vi "ZLIB File Information__ogtk.vi"(0 "file path":path, 1 "encode MacBinary (F)":bool, 3 "error in (no error)":errorcluster) -> (4 "created macbinary":bool, 5 "file timestamp":u32, 6 "file path out":path, 7 "directory":bool, 8 "file attributes":u32, 9 "error out":errorcluster)   [LabVIEW 2011]
doc: "Retrives specific information for a disk file preparing a Mac resource files as MACBIN data file fork."
panel:
  # "Please visit http://www.OpenG.org to learn about the\nOpen Source LabVIEW software movement.\n\nNOTICE -- YOU MUST LEAVE THIS NOTICE IN PLACE.  PER THE TERMS OF THE LICENSE BELOW, YOU MAY SUBLICENSE THIS SOFTWARE \nIN ANY WAY THAT DOES NOT CONFLICT WITH THIS LICENSE.\n\n### BSD License (http://www.opensource.org/licenses/bsd-license.php) Begin ###\n \nCopyright (C) 2008 Rolf Kalbermatter rolf.kalbermatter@citeng.com\n\nAll rights reserved.\n\nRedistribution and use in source and binary forms, with or without modification, are permitted provided that the following conditions are met:\n\n    * Redistributions of source code must retain the above copyright notice, this list of conditions and the following disclaimer.\n    * Redistributions in binary form must reproduce the above copyright notice, this list of conditions and the following disclaimer in the \n       documentation and/or other materials provided with the distribution.\n    * Neither the name of SciWare, James Kring, Inc., nor the names of its contributors may be used to endorse or promote products derived \n       from this software without specific prior written permission.\n\nTHIS SOFTWARE IS PROVIDED BY THE COPYRIGHT HOLDERS AND CONTRIBUTORS \"AS IS\" AND ANY EXPRESS OR IMPLIED WARRANTIES, \nINCLUDING, BUT NOT LIMITED TO, THE IMPLIED WARRANTIES OF MERCHANTABILITY AND FITNESS FOR A PARTICULAR PURPOSE ARE \nDISCLAIMED. IN NO EVENT SHALL THE COPYRIGHT OWNER OR CONTRIBUTORS BE LIABLE FOR ANY DIRECT, INDIRECT, INCIDENTAL,\n SPECIAL, EXEMPLARY, OR CONSEQUENTIAL DAMAGES (INCLUDING, BUT NOT LIMITED TO, PROCUREMENT OF SUBSTITUTE GOODS OR \nSERVICES; LOSS OF USE, DATA, OR PROFITS; OR BUSINESS INTERRUPTION) HOWEVER CAUSED AND ON ANY THEORY OF LIABILITY, \nWHETHER IN CONTRACT, STRICT LIABILITY, OR TORT (INCLUDING NEGLIGENCE OR OTHERWISE) ARISING IN ANY WAY OUT OF THE USE \nOF THIS SOFTWARE, EVEN IF ADVISED OF THE POSSIBILITY OF SUCH DAMAGE.\n\n### BSD License End ###"
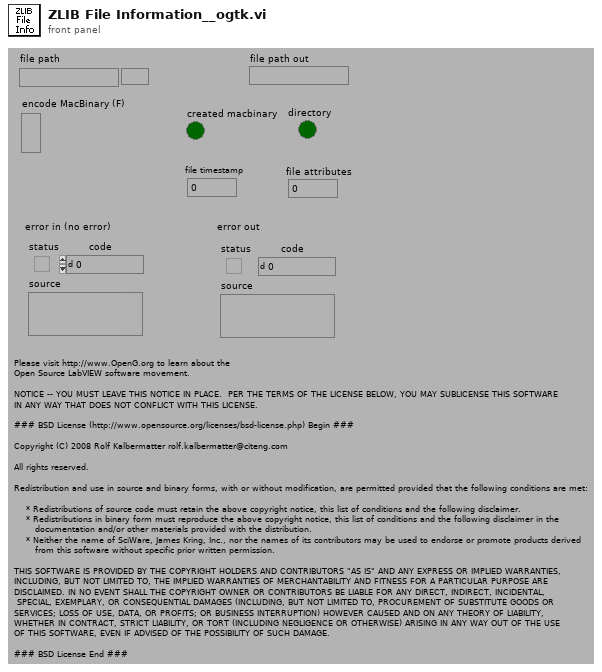
[diagram p1: front panel]
types:
  T1 = typedef "MACBIN Resource Header__ogtk.ctl" = cluster{"type":string, "creator":string, "data size":u32, "res size":u32, "creation date":u32, "mod date":u32, "finder flags":u16, "vertical pos":i16, "horizontal pos":i16, "finder id":u16, "script id":u8, "ext finder flags":u8}
  T2 = typedef "Librarian File Info Out.ctl" = cluster{"creation date":u32, "last mod date":u32, "type":string, "creator":string, "LV version":i32, "size":i32, "top level":bool}
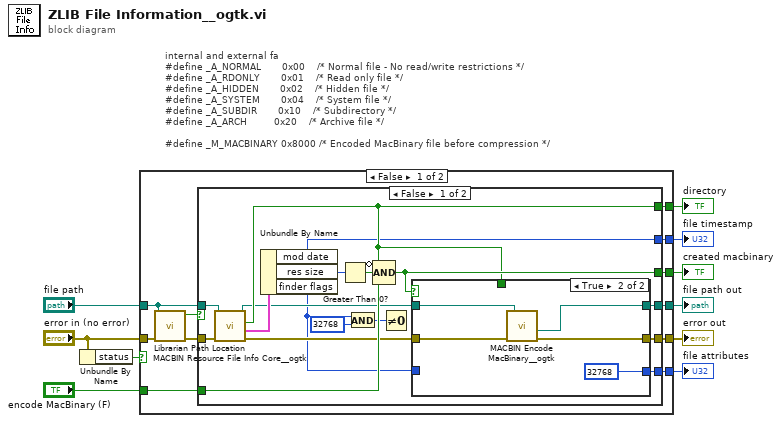
[diagram p0: block diagram]
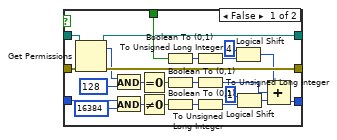
[diagram p2: hidden frame]
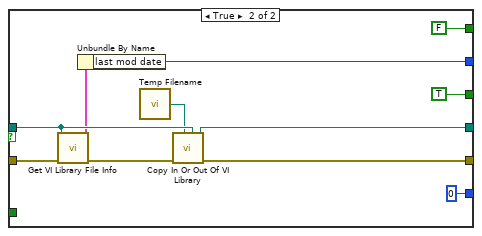
[diagram p3: hidden frame]
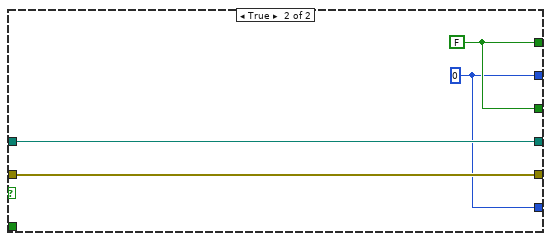
[diagram p4: hidden frame]
diagram:
  # "internal and external fa\n#define _A_NORMAL       0x00    /* Normal file - No read/write restrictions */\n#define _A_RDONLY       0x01    /* Read only file */\n#define _A_HIDDEN       0x02    /* Hidden file */\n#define _A_SYSTEM       0x04    /* System file */\n#define _A_SUBDIR       0x10    /* Subdirectory */\n#define _A_ARCH         0x20    /* Archive file */\n\n#define _M_MACBINARY 0x8000 /* Encoded MacBinary file before compression */"
  n1 = Unbundle By Name("error in (no error)") -> ("status"=w3:bool)
  n2 = case shown="False" w3 {
    tunnel: "file path" -> [w11 w82]
    tunnel: [w15 w79] -> w9
    tunnel: [w16 w80] -> w8
    tunnel: "error in (no error)" -> [w14 w81]
    tunnel: [w21 w82] -> w6
    tunnel: [w20 w81] -> w5
    tunnel: [w19 w79] -> w4
    tunnel: [w18 w80] -> w2
    tunnel: "encode MacBinary (F)" -> [w17 _]
    frame False {
      n3 = call <vilib>:"Librarian Path Location.vi"("error in (no error)"=w14, "path"=w11) -> ("error out"=w13:errorcluster, "path is in a VI library"=w12:bool)  [unwired: 5 in, 3 out]
      n4 = case shown="False" w12 {
        tunnel: w13 -> [w38 w77]
        tunnel: [w37 w71] -> w21
        tunnel: [w36 w72] -> w20
        tunnel: [w35 u32 0 ("Input")] -> w19
        tunnel: [w34 TRUE] -> w18
        tunnel: w17 -> [w33 _]
        tunnel: w11 -> [w32 w76]
        tunnel: [w31 FALSE ("is directory")] -> w16
        tunnel: [w29 w73] -> w15
        frame False {
          n5 = call <userlib>:"MACBIN Resource File Info Core__ogtk.vi"("error in (no error)"=w38, "resource file"=w32) -> ("error out"=w25:errorcluster, "file info out"=w30:T1, "is directory"=w31:bool, "resource file out"=w26:path)  [unwired: 3 in, 1 out]
          n6 = Unbundle By Name(w30) -> ("mod date"=w29:u32, "res size"=w28:u32, "finder flags"=w24:u16)
          n7 = Greater Than 0?(x=w28) -> (x > 0?=w27:bool)
          n8 = And(x=w24, y=u16 32768) -> (x .and. y?=w22:u16)
          n9 = Compound Arithmetic op=AND(invert w31, w27, w33) -> (w34:bool)
          n10 = Not Equal To 0?(x=w22) -> ()  [unwired: 1 out]
          n11 = case shown="True" w34 {
            tunnel: [w55 w67] -> w37
            tunnel: [w54 w66] -> w36
            tunnel: w26 -> [w56 w64]
            tunnel: w25 -> [w57 w63]
            tunnel: [w62 u32 32768 ("Input")] -> w35
            tunnel: w31 -> [w59 _]
            tunnel: w24 -> [w46 _]
            frame False {
              n12 = Get Permissions(8:w57, 11:w56) -> (0:w54:errorcluster, 3:w55:path, 5:w49:i16)  [unwired: 2 out]
              n13 = And(x=w49, y=i16 128) -> (x .and. y?=w53:i16)
              n14 = And(x=w46, y=u16 16384) -> (x .and. y?=w48:u16)
              n15 = Equal To 0?(x=w53) -> (x = 0?=w52:bool)
              n16 = Not Equal To 0?(x=w48) -> (x != 0?=w58:bool)
              n17 = Boolean To (0,1)(Boolean=w59) -> (0, 1=w41:i16)
              n18 = Boolean To (0,1)(Boolean=w52) -> (0, 1=w50:i16)
              n19 = Boolean To (0,1)(Boolean=w58) -> (0, 1=w45:i16)
              n20 = To Unsigned Long Integer(number=w41) -> (unsigned 32bit integer=w40:u32)
              n21 = To Unsigned Long Integer(number=w50) -> (unsigned 32bit integer=w43:u32)
              n22 = To Unsigned Long Integer(number=w45) -> (unsigned 32bit integer=w44:u32)
              n23 = Logical Shift(y=i16 4, x=w40) -> (x << y=w39:u32)
              n24 = Logical Shift(y=i16 1, x=w44) -> (x << y=w42:u32)
              n25 = Compound Arithmetic op=ADD(w39, w43, w42) -> (w62:u32)
            }
            frame True {
              n26 = call <userlib>:"MACBIN Encode MacBinary__ogtk.vi"("error in (no error)"=w63, "data file"=w64) -> ("error out"=w66:errorcluster, "macbinary file out"=w67:path)  [unwired: 2 in, 2 out]
            }
          }
        }
        frame True {
          n27 = call <vilib>:"Get VI Library File Info.vi"("error in (no error)"=w77, "path"=w76) -> ("error out"=w75:errorcluster, "file information"=w74:T2)  [unwired: 8 in]
          n28 = Unbundle By Name(w74) -> ("last mod date"=w73:u32)
          n29 = call <vilib>:"Temp Filename.vi"() -> ("file in tmp dir"=w69:path)
          n30 = call <vilib>:"Copy In Or Out Of VI Library.vi"("source"=w76, "destination"=w69, "error in (no error)"=w75) -> ("error out"=w72:errorcluster, "dup destination"=w71:path)  [unwired: 7 in]
        }
      }
    }
    frame True {
      w79 = u32 0 ("mod date")
      w80 = FALSE ("directory")
    }
  }
  "file timestamp" <- w9
  "directory" <- w8
  "error out" <- w5
  "file path out" <- w6
  "file attributes" <- w4
  "created macbinary" <- w2
